vi "Select Cell.vi"(8 "error in (no error)":errorcluster, 10 "Index selector":i32=-1, 11 "Run Block in":refnum<class "Run Block.lvclass">) -> (0 "error out":errorcluster, 3 "Run Block out":refnum<class "Run Block.lvclass">)   [LabVIEW 2020, in "Run Utilities.lvlib" / "Run Block.lvclass"]
doc: "This VI does a check if the index is in the range <-1,schedule size) and it coerces index to the min/max values. This VI is the backend of the <b>Write Index selector Property Node</b>."
uses:
  Run Block.lvclass
  Run Block.lvclass/Run Block.ctl
  Schedule/Schedule.lvclass
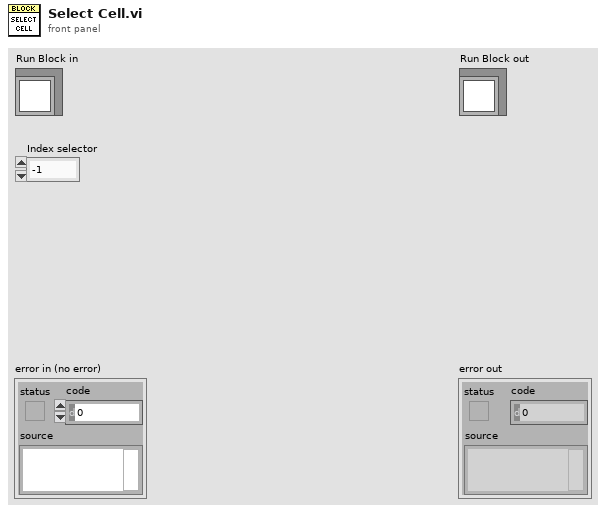
[diagram p1: front panel]
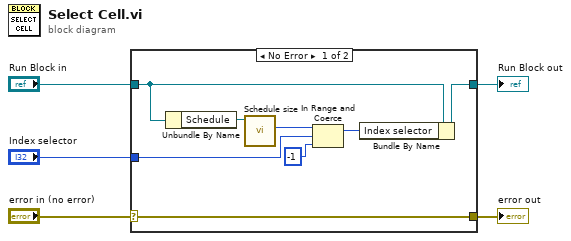
[diagram p0: block diagram]
diagram:
  n1 = case shown="No Error" "error in (no error)" {
    selector: "error in (no error)" -> [w13 w14]
    tunnel: [w13 w14] -> w4
    tunnel: [w12 w15] -> w2
    tunnel: "Run Block in" -> [w11 w15]
    tunnel: "Index selector" -> [w7 _]
    frame No Error {
      n2 = Unbundle By Name(w11) -> ("Schedule"=w10:refnum<class "Schedule.lvclass">)
      n3 = call-dynamic "Schedule size.vi"("Schedule in"=w10) -> ("Size"=w8:i32)  [unwired: 8 in, 2 out]
      n4 = In Range and Coerce(upper limit=w8, x=w7, lower limit=-1 ("t")) -> (coerced(x)=w6:i32)  [unwired: 1 out]
      n5 = Bundle By Name(cluster=w11, "Index selector"=w6) -> (w12:refnum<class "Run Block.lvclass">)
    }
    frame Error {
    }
  }
  "error out" <- w4
  "Run Block out" <- w2
